vi "My SIM PID.vi"(0 "Setpoint":dbl, 1 "Measurement":dbl, 2 "Tracking":dbl, 3 "Integral antiwindup [s] (Ti)":dbl=1.0, 4 "Setpoint weighting (Beta)":dbl, 5 "Setpoint weighting (Gamma)":dbl, 6 "Initialize?":bool, 7 "Proportional Gain (Kc)":dbl=1.0, 8 "Tracking?":bool, 9 "Integral time [s] (Ti)":dbl=1.0, 10 "Auto?":bool, 11 "Derivative time [s] (Td)":dbl=1.0, 12 "Manual":dbl, 13 "High Frequency [s] (Tf)":dbl=1.0, 14 "output range":cluster{"output high":dbl, "output low":dbl}={"output high"=inf, "output low"=-inf} {"output low" format="%.2f"; "output high" format="%.2f"}) -> (17 "Output":dbl)   [LabVIEW 2012]
uses:
  <vilib>/Simulation/Model Libraries/PID/subVIs/SIM PID Integral Gain.vi
  My SIM PID Derivative Gain.vi
  <vilib>/Simulation/Implementation/Shared/SIMSCR Execution Mode.ctl
  <vilib>/Simulation/Scripting/Companion Diagram/SimConfigNode/SimParams.ctl
  <vilib>/Simulation/Scripting/Companion Diagram/SimConfigNode/_simSolvers.ctl
  <vilib>/Simulation/Param Hierarchy/Typedefs/SIMPH Param Control Actions.ctl
  <vilib>/Simulation/Implementation/Shared/NILVSim_ParamChanged.vi
  <vilib>/Simulation/SignalArithmetic/Implementation/NILVSim Gain.llb/SIM Gain (scalar).vi
  <vilib>/Simulation/Nonlinear/Implementation/NILVSim Saturation.llb/SIM Saturation (scalar).vi
  <vilib>/Simulation/Implementation/Shared/NILVSim_Manager.vi
  <vilib>/Simulation/Implementation/Shared/NILVSim_FinalizeModel.vi
  <vilib>/Simulation/Implementation/Shared/SIM Unbundle Sim Info.vi
  <vilib>/Utility/error.llb/Clear Errors.vi
  <vilib>/Simulation/Implementation/Shared/NILVSim_GetModelError.vi
  <vilib>/Simulation/Implementation/Shared/SIM SimErrorHandler.vi
  <vilib>/Simulation/Implementation/Shared/SIM Bundle Sim Info.vi
  <vilib>/Simulation/Implementation/Shared/NILVSim_Initialize.vi
  <vilib>/Simulation/Utility/Implementation/NILVSim Get Time and IsAcceptedStep.vi
  <vilib>/Simulation/Implementation/Shared/SIMSH Read Queue.vi
  <vilib>/Simulation/Scripting/Companion Diagram/SimConfigNode/SimDog.xnode
  <vilib>/Simulation/Implementation/XNodeFramework/SimXNode/SimX.xnode
  <vilib>/Simulation/Implementation/Shared/NI_SIM_Implementation.lvlib
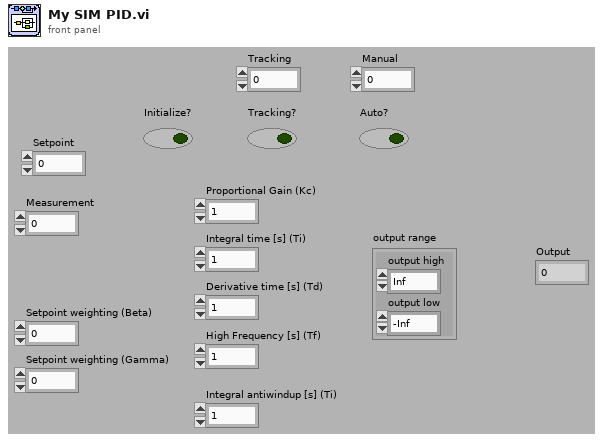
[diagram p1: front panel]
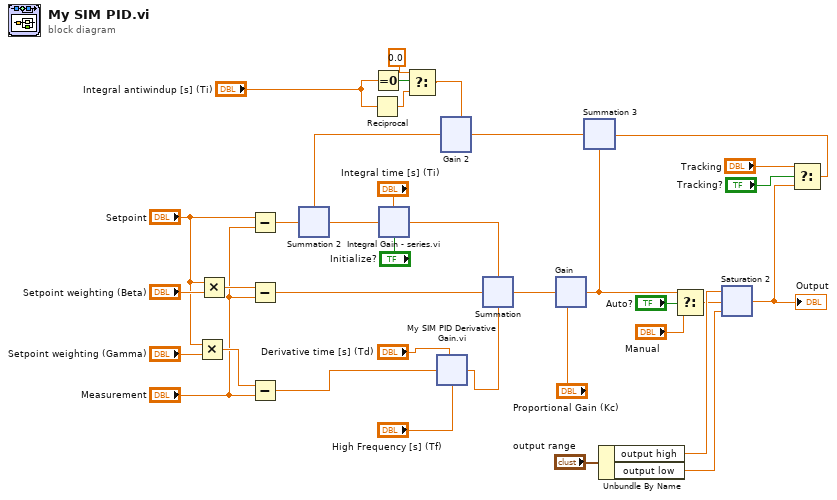
[diagram p0: block diagram]
diagram:
  n1 = Multiply ("Multiply 2")(x="Setpoint", y="Setpoint weighting (Gamma)") -> (x*y=w30:dbl)
  n2 = Multiply(x="Setpoint", y="Setpoint weighting (Beta)") -> (x*y=w32:dbl)
  n3 = Subtract ("Subtract 3")(x="Setpoint", y="Measurement") -> (x-y=w25:dbl)
  n4 = Subtract(x=w32, y="Measurement") -> (x-y=w29:dbl)
  n5 = Subtract ("Subtract 2")(x=w30, y="Measurement") -> (x-y=w3:dbl)
  n6 = Reciprocal(x="Integral antiwindup [s] (Ti)") -> (1/x=w13:dbl)
  n7 = Equal To 0?(x="Integral antiwindup [s] (Ti)") -> (x = 0?=w14:bool)
  n8 = Select ("Select 3")(t=0.0, s=w14, f=w13) -> (s? t:f=w10:dbl)
  n9 = xnode "My SIM PID Derivative Gain.vi"("Derivative Gain"="Derivative time [s] (Td)", "Error"=w3, "High Frequency [s] (Tf)"="High Frequency [s] (Tf)") -> ("output"=w2:dbl)  [unwired: 12 out]
  n10 = Unbundle By Name("output range") -> ("output high"=w7:dbl, "output low"=w8:dbl)
  n11 = xnode ("Summation 2")("Operand1"=w22, "Operand2"=w25) -> ("Result"=w24:dbl)
  n12 = xnode ("Integral Gain - series.vi")("Integral Gain"="Integral time [s] (Ti)", "Error"=w24, "reset?"="Initialize?") -> ("output"=w26:dbl)  [unwired: 1 in, 11 out]
  n13 = xnode ("Summation")("Operand1"=w26, "Operand2"=w29, "Operand3"=w2) -> ("Result"=w36:dbl)
  n14 = xnode ("Gain")("gain"="Proportional Gain (Kc)", "input"=w36) -> ("output"=w19:dbl)  [unwired: 2 in]
  n15 = Select(t=w19, s="Auto?", f="Manual") -> (s? t:f=w6:dbl)
  n16 = xnode "Saturation 2"("upper limit"=w7, "input"=w6, "lower limit"=w8) -> ("output"=w5:dbl)  [unwired: 2 in]
  "Output" <- w5
  n17 = Select ("Select 2")(t="Tracking", s="Tracking?", f=w5) -> (s? t:f=w16:dbl)
  n18 = xnode ("Summation 3")("Operand1"=w16, "Operand2"=w19) -> ("Result"=w23:dbl)
  n19 = xnode ("Gain 2")("gain"=w10, "input"=w23) -> ("output"=w22:dbl)  [unwired: 2 in]
